vi "PlotObjectArray_get_and_lock.vi"(7 "External PlotObjQueue in":refnum<queue>, 8 "error in (no error)":errorcluster) -> (0 "error out":errorcluster, 3 "PlotObjects":refnum<class "Plots.lvclass">[](array[class]))   [LabVIEW 2017]
doc: "the VI locks and returns/reads the PlotObjectsArray using a Queue.\n\nExternal PlotObjQueue is only needed when called from MSEval!!!"
uses:
  Classes/Plots/Plots.lvclass
  global variables.vi
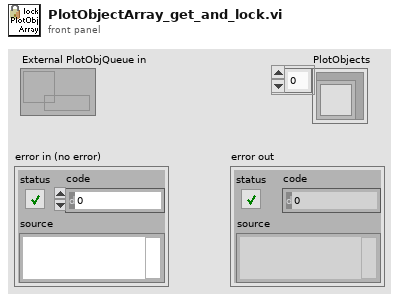
[diagram p1: front panel]
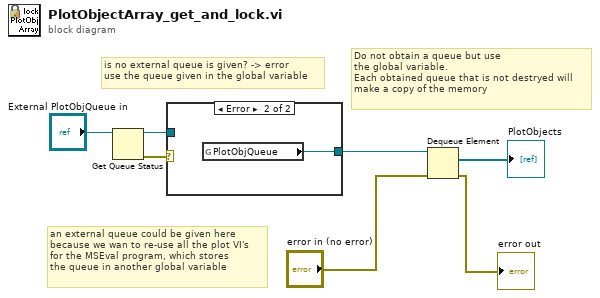
[diagram p0: block diagram]
diagram:
  # "an external queue could be given here\nbecause we wan to re-use all the plot VI's\nfor the MSEval program, which stores\nthe queue in another global variable"
  # "is no external queue is given? -> error\nuse the queue given in the global variable"
  # "Do not obtain a queue but use\nthe global variable.\nEach obtained queue that is not destryed will\nmake a copy of the memory"
  n1 = Get Queue Status(queue="External PlotObjQueue in") -> (queue out=w1:refnum<queue>, error out=w2:errorcluster)  [unwired: 2 in, 6 out]
  n2 = case shown="Error" w2 {
    tunnel: [w8 w9] -> w6
    tunnel: w1 -> [w8 _]
    frame No Error {
    }
    frame Error {
      n3 = global read "global variables.vi" "PlotObjQueue"() -> (w9:refnum<queue>)
    }
  }
  n4 = Dequeue Element(queue=w6, error in (no error)="error in (no error)") -> (element=→"PlotObjects":refnum<class "Plots.lvclass">[], error out=→"error out":errorcluster)  [unwired: 1 in, 2 out]
